vi "Untitled 1.vi"() -> ()   [LabVIEW 2021, in "Test VIs.lvclass"]
uses:
  Test VIs/Test VIs.lvclass
  Classes/Controller/Controller.lvclass
  Classes/Controller/Dispenser/Dispenser.lvclass
panel:
  in  "stop":bool
  in  "dispense":bool
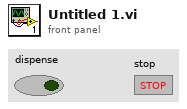
[diagram p1: front panel]
types:
  T1 = typedef "Controller.lvclass/Controllers.ctl" = cluster{"I-O.lvclass":refnum<class "I-O.lvclass">, "Gantry":refnum<k24>, "Dispenser":refnum<visa-resource-name>}
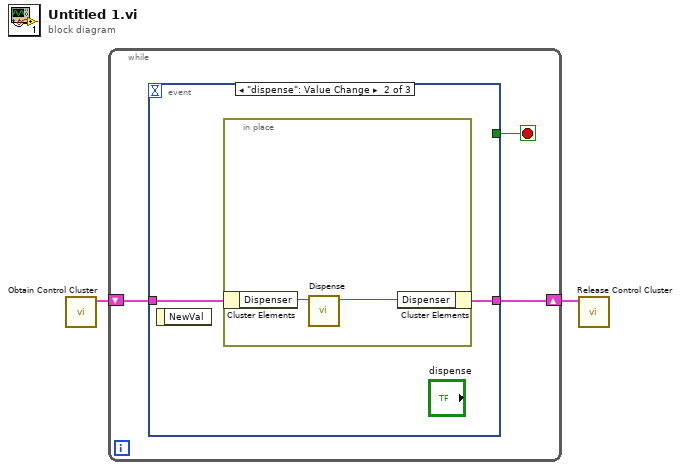
[diagram p0: block diagram]
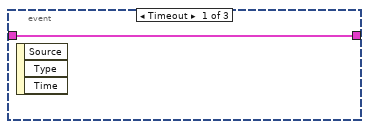
[diagram p2: hidden frame]
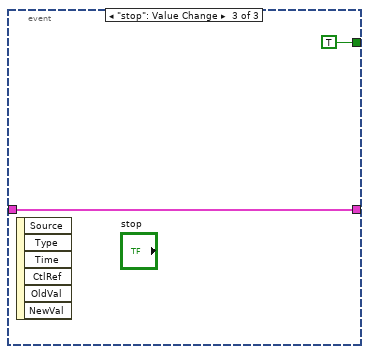
[diagram p3: hidden frame]
diagram:
  n1 = call "Obtain Control Cluster.vi"() -> ("Control Out"=w2:T1)  [unwired: 10 in, 1 out]
  n2 = while {
    shift-right: [w4] -> w1
    shift-left: w2 -> [w5]
    stop <- w3 stop-if-true
    n3 = event shown="[1] \"dispense\": Value Change" {
      selector: _ -> [_ _ _]
      dyn-events: _ -> [_ _ _]
      timeout: _ -> [_ _ _]
      tunnel: w5 -> [w6 w8 w11]
      tunnel: [w6 w7 w11] -> w4
      tunnel: [_ _ TRUE] -> w3
      event Timeout {
        n4 = event-data() -> ()  [unwired: 1 in, 3 out]
      }
      event "dispense": Value Change {
        n5 = event-data() -> ()  [unwired: 1 in, 1 out]
        n6 = in-place {
          n7 = in-place-cluster #1(w8) -> ("Dispenser"=w10:refnum<visa-resource-name>)
          n8 = call "Dispense.vi"("Dispenser In"=w10) -> ("Dispenser Out"=w9:refnum<visa-resource-name>)  [unwired: 9 in, 1 out]
          n9 = in-place-cluster #1("Dispenser"=w9) -> (w7:T1)
        }
      }
      event "stop": Value Change {
        n10 = event-data() -> ()  [unwired: 1 in, 6 out]
      }
    }
  }
  n11 = call "Release Control Cluster.vi"("output cluster"=w1) -> ()  [unwired: 11 in]
